vi "SSC Digital Filter Sites.vi"(0 "Digital SSC In":T1[](array[typedef]), 5 "Desired Sites":i32[](array[numeric]), 11 "error in":errorcluster) -> (4 "Digital SSC Out with requested sites":T1[](array[typedef]), 15 "error out":errorcluster)   [LabVIEW 2019]
doc: "Filters Digital SSC sessions based on the specified list of desired sites. \n\nNOTE: Once sessions have been filtered, they become separated from their original TSM context and cannot be properly published using pin query context."
uses:
  SSC Digital.ctl
  Shared SubVIs/Site List to Site Numbers.vi
  Shared SubVIs/Channel List to Pins.vi
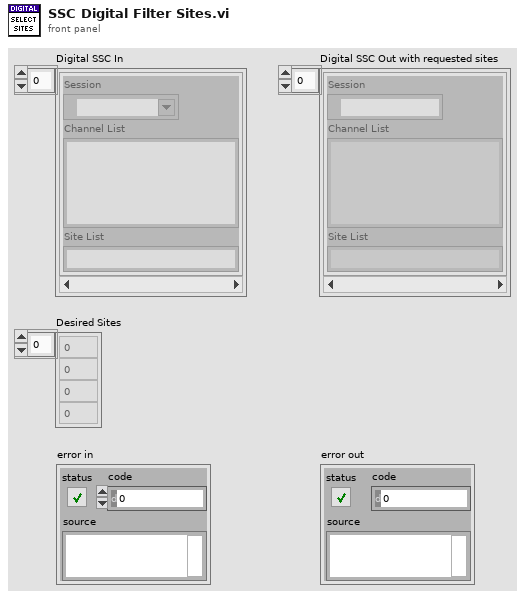
[diagram p1: front panel]
types:
  T1 = typedef "SSC Digital.ctl" = cluster{"Session":refnum<k15>, "Channel List":string, "Site List":string}
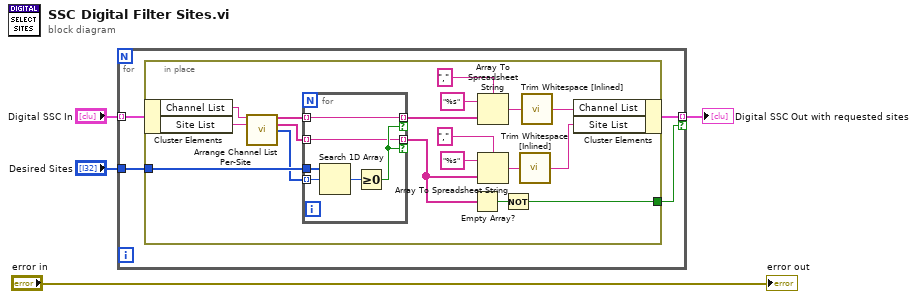
[diagram p0: block diagram]
diagram:
  n1 = for {
    tunnel: "Digital SSC In" -> [w8] mode=indexing
    tunnel: "Desired Sites" -> [w5]
    tunnel: [w7] -> w2 mode=indexing if=w6
    n2 = in-place {
      in-place-border: w5 -> [w24]
      in-place-border: [w10] -> w6
      n3 = in-place-cluster #1(w8) -> ("Channel List"=w26:string, "Site List"=w25:string)
      n4 = call "Arrange Channel List Per-Site.vi"("Channel List String"=w26, "Site List String"=w25) -> ("Channel List Array"=w22:string[], "Site List Array"=w21:string[], "Site Numbers"=w23:i32[])  [unwired: 11 in]
      n5 = for {
        tunnel: w22 -> [w30] mode=indexing
        tunnel: w23 -> [w29] mode=indexing
        tunnel: w24 -> [w32]
        tunnel: [w30] -> w12 mode=indexing if=w28
        tunnel: [w27] -> w9 mode=indexing if=w28
        tunnel: w21 -> [w27] mode=indexing
        n6 = Search 1D Array(1D array=w32, element=w29) -> (index of element=w31:i32)  [unwired: 1 in]
        n7 = Greater Or Equal To 0?(x=w31) -> (x >= 0?=w28:bool)
      }
      n8 = Empty Array?(array=w9) -> (empty?=w11:bool)
      n9 = Array To Spreadsheet String(delimiter (Tab)=",", array=w12, 3:"%s" ("format string")) -> (spreadsheet string=w16:string)
      n10 = Array To Spreadsheet String(delimiter (Tab)=",", array=w9, 3:"%s" ("format string")) -> (spreadsheet string=w14:string)
      n11 = Not(x=w11) -> (.not. x?=w10:bool)
      n12 = call "Trim Whitespace [Inlined].vi"("string"=w14) -> ("trimmed string"=w13:string)  [unwired: 1 in]
      n13 = call "Trim Whitespace [Inlined].vi"("string"=w16) -> ("trimmed string"=w15:string)  [unwired: 1 in]
      n14 = in-place-cluster #1("Channel List"=w15, "Site List"=w13) -> (w7:T1)
    }
  }
  "Digital SSC Out with requested sites" <- w2
  "error out" <- "error in"
